vi "主程序.vi"() -> ()   [LabVIEW 2010]
panel:
  out "loop number":dbl
  in  "?":bool
  out "number:0 to 1":dbl
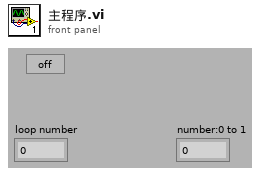
[diagram p1: front panel]
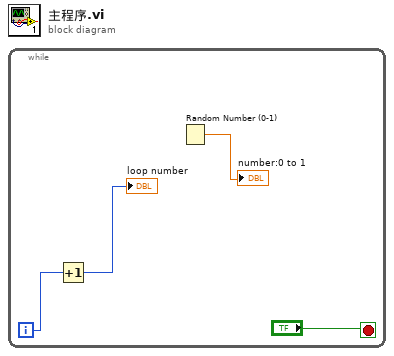
[diagram p0: block diagram]
diagram:
  n1 = while {
    i -> [w2]
    stop <- "?" stop-if-true
    n2 = Increment(x=w2) -> (x+1=→"loop number":i32)
    n3 = Random Number (0-1)() -> (number: 0 to 1=→"number:0 to 1":dbl)
  }
